vi "Decorate Core Actor.vi"(4 "Stop When Parent Stopped":bool=TRUE, 10 "Actor To Decorate Core Actor":refnum<class "Actor.lvclass">) -> (2 "Decorated Core Actor":refnum<class "Actor.lvclass">)   [LabVIEW 2025, in "jettl.lvlib" / "Actor.lvlib"]
uses:
  Actor.lvlib
  Actor/Actor.lvclass
  Core Actor/Core Actor.lvclass
  C:/git/jettl/src/jettl/jettl/Actor/Actor/Actor.lvclass
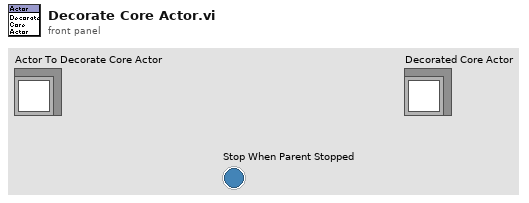
[diagram p1: front panel]
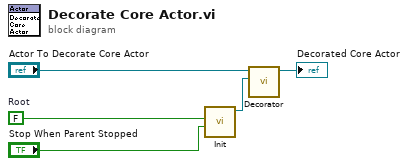
[diagram p0: block diagram]
diagram:
  w2 = FALSE  # Root
  n1 = call "Init.vi"("Stop When Parent Stopped"="Stop When Parent Stopped", "Root"=w2) -> ("Core Actor out"=w5:refnum<class "Core Actor.lvclass">)  [unwired: 9 in]
  n2 = call-dynamic "Decorator.vi"("Actor"=w5, "Actor in"="Actor To Decorate Core Actor") -> ("Actor out"=→"Decorated Core Actor":refnum<class "Actor.lvclass">)  [unwired: 9 in]
